vi "User Interface.vi"(8 "error in (no error)":errorcluster, 11 "User Interface in":refnum<class "User Interface.lvclass">) -> (0 "error out":errorcluster, 3 "User Interface out":refnum<class "User Interface.lvclass">)   [LabVIEW 2017, in "DSF Core.lvlib" / "Component Settings Editor.lvclass"]
uses:
  Component Settings Editor.lvclass
  User Interface.lvclass
  C:/Git/DSF/Core/Classes/User Interface/User Interface.lvclass
  Component Settings Editor.lvclass/Component Settings Editor.ctl
  User Interface Handler/User Interface Handler.lvclass
panel:
  in  "Components":i32(listbox)
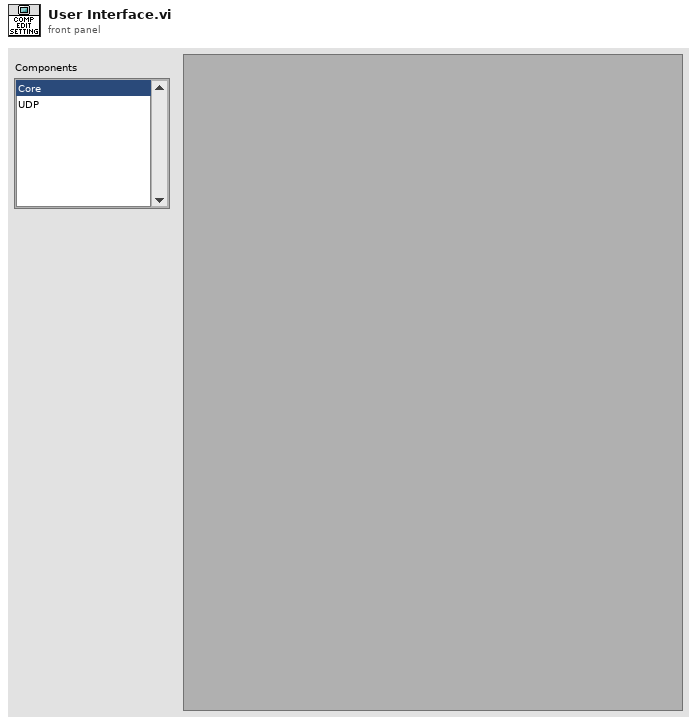
[diagram p1: front panel]
types:
  T1 = typedef "DSF Core.lvlib/User Interface Handler.lvclass/User Interface Ref.ctl" = refnum<vi>
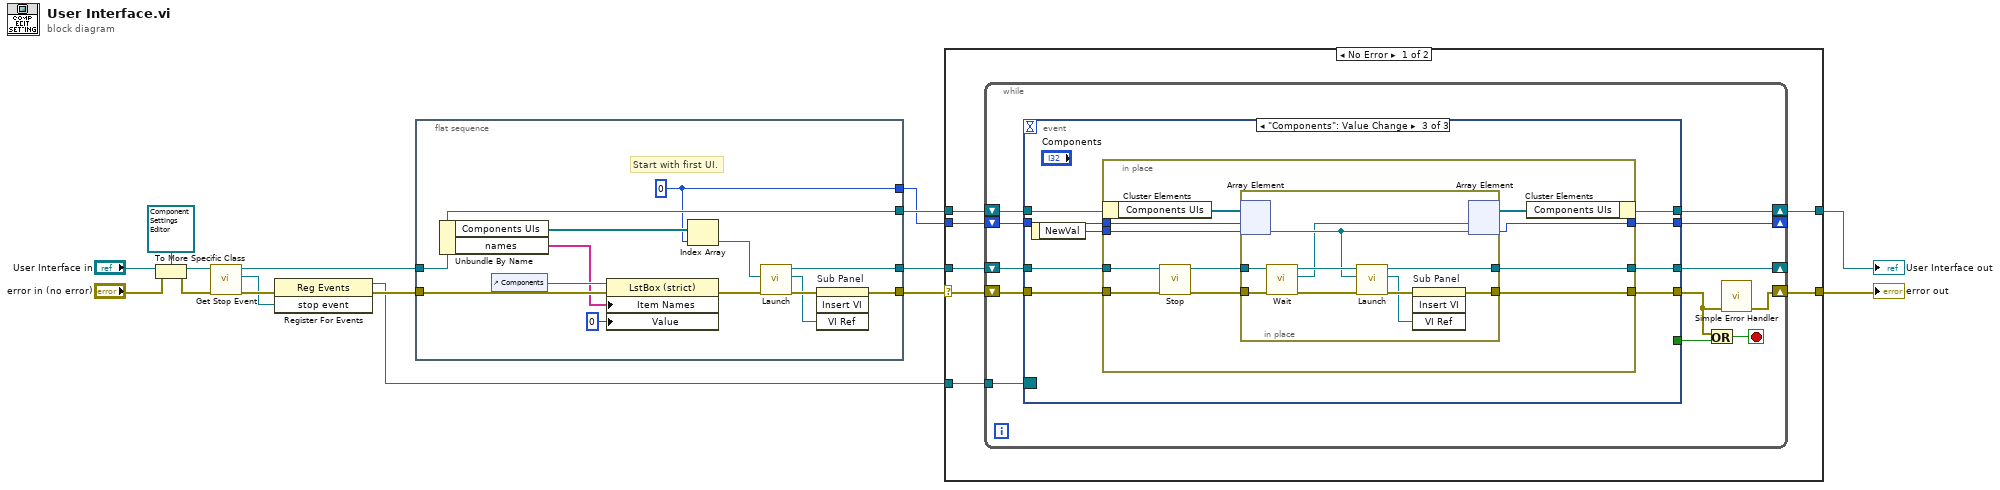
[diagram p0: block diagram]
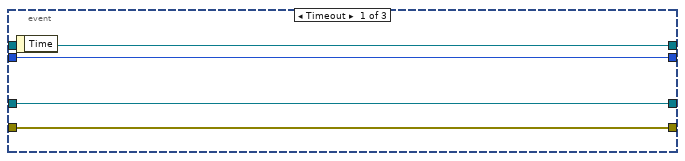
[diagram p2: hidden frame]
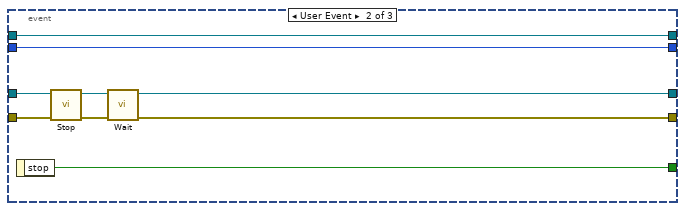
[diagram p3: hidden frame]
diagram:
  n1 = To More Specific Class(target class=refnum<class "Component Settings Editor.lvclass"> refnum ("DSF Core.lvlib:Plugin Settings Editor.lvclass"), reference="User Interface in", error in="error in (no error)") -> (specific class reference=w10:refnum<class "Component Settings Editor.lvclass">, error out=w9:errorcluster)
  n2 = call "Get Stop Event.vi"("error in (no error)"=w9, "User Interface in"=w10) -> ("error out"=w12:errorcluster, "stop event"=w11:refnum<user-event>, "User Interface out"=w4:refnum<class "Component Settings Editor.lvclass">)  [unwired: 7 in]
  n3 = register-events(error in=w12, w11) -> (reference out=w6:refnum<event-registration>, error out=w7:errorcluster)  [unwired: 1 in]
  n4 = flat-sequence {
    tunnel: w7 -> [w28]
    tunnel: [w25] -> w1
    tunnel: [w23] -> w5
    tunnel: w4 -> [w22]
    tunnel: [w22] -> w3
    tunnel: [w17] -> w2
    frame #0 {
      w17 = 0
      # "Start with first UI."
      n5 = Unbundle By Name(w22) -> ("Components UIs"=w21:refnum<class "User Interface.lvclass">[], "names"=w20:string[])
      n6 = control-ref of="Components"() -> (w29:refnum<vi>)
      n7 = property class="LstBox (strict)"(reference=w29, error in=w28, "Item Names"=w20, "Value"=0) -> (error out=w18:errorcluster)  [unwired: 1 out]
      n8 = Index Array(array=w21, index=w17) -> (element=w19:refnum<class "User Interface.lvclass">)
      n9 = call "Launch.vi"("error in (no error)"=w18, "User Interface"=w19) -> ("error out"=w26:errorcluster, "active vi"=w24:T1, "User Interface Handler out"=w23:refnum<class "User Interface Handler.lvclass">)  [unwired: 7 in]
      n10 = invoke on="Sub Panel" class="SubPnl" method="Insert VI"(error in=w26, "VI Ref"=w24) -> (error out=w25:errorcluster)  [unwired: 2 in, 3 out]
    }
  }
  n11 = case shown="No Error" w1 {
    selector: w1 -> [w30 w93]
    tunnel: [w36 w93] -> w16
    tunnel: [w35 w92] -> w13
    tunnel: w6 -> [w34 _]
    tunnel: w5 -> [w33 _]
    tunnel: w3 -> [w32 w92]
    tunnel: w2 -> [w31 _]
    frame No Error {
      n12 = while {
        tunnel: w34 -> [w48]
        shift-right: [w37] -> w36
        shift-left: w30 -> [w47]
        shift-right: [w43] -> _
        shift-left: w33 -> [w44]
        shift-right: [w41] -> w35
        shift-left: w32 -> [w42]
        shift-right: [w39] -> _
        shift-left: w31 -> [w40]
        stop <- w46 stop-if-true
        n13 = event shown="[2] \"Components\": Value Change" {
          selector: w48 -> [_ _ _]
          dyn-events: _ -> [_ _ _]
          timeout: _ -> [_ _ _]
          tunnel: [_ w61 _] -> w45
          tunnel: w47 -> [w52 w57 w65]
          tunnel: [w52 w56 w62] -> w38
          tunnel: w44 -> [w51 w58 w64]
          tunnel: [w51 w55 w63] -> w43
          tunnel: w42 -> [w50 w54 w70]
          tunnel: [w50 w54 w69] -> w41
          tunnel: w40 -> [w49 w53 w67]
          tunnel: [w49 w53 w66] -> w39
          event Timeout {
            n14 = event-data() -> ()  [unwired: 1 in, 1 out]
          }
          event User Event {
            n15 = event-data() -> ("stop"=w61:bool)  [unwired: 1 in]
            n16 = call "Stop.vi"("error in (no error)"=w57, "User Interface Handler in"=w58) -> ("error out"=w59:errorcluster, "User Interface Handler out"=w60:refnum<class "User Interface Handler.lvclass">)  [unwired: 8 in]
            n17 = call "Wait.vi"("error in (no error)"=w59, "User Interface Handler in"=w60) -> ("error out"=w56:errorcluster, "User Interface Handler out"=w55:refnum<class "User Interface Handler.lvclass">)  [unwired: 7 in, 1 out]
          }
          event "Components": Value Change {
            n18 = event-data() -> ("NewVal"=w68:i32)  [unwired: 1 in]
            n19 = in-place {
              in-place-border: w67 -> [w81]
              in-place-border: w68 -> [w77]
              in-place-border: [w80] -> w66
              in-place-border: w65 -> [w73]
              in-place-border: w64 -> [w74]
              in-place-border: [w79] -> w63
              in-place-border: [w78] -> w62
              n20 = in-place-cluster #1(w70) -> ("Components UIs"=w76:refnum<class "User Interface.lvclass">[])
              n21 = call "Stop.vi"("error in (no error)"=w73, "User Interface Handler in"=w74) -> ("error out"=w72:errorcluster, "User Interface Handler out"=w71:refnum<class "User Interface Handler.lvclass">)  [unwired: 8 in]
              n22 = in-place {
                in-place-border: [w89] -> w79
                in-place-border: [w90] -> w78
                in-place-border: w72 -> [w83]
                in-place-border: w71 -> [w82]
                n23 = in-place-array #2(w76, w81, w77) -> (w85:refnum<class "User Interface.lvclass">)  [unwired: 1 out]
                n24 = call "Wait.vi"("error in (no error)"=w83, "User Interface Handler in"=w82) -> ("error out"=w87:errorcluster, "User Interface"=w84:refnum<class "User Interface.lvclass">, "User Interface Handler out"=w86:refnum<class "User Interface Handler.lvclass">)  [unwired: 7 in]
                n25 = call "Launch.vi"("error in (no error)"=w87, "User Interface"=w85, "User Interface Handler in"=w86) -> ("error out"=w91:errorcluster, "active vi"=w88:T1, "User Interface Handler out"=w89:refnum<class "User Interface Handler.lvclass">)  [unwired: 6 in]
                n26 = invoke on="Sub Panel" class="SubPnl" method="Insert VI"(error in=w91, "VI Ref"=w88) -> (error out=w90:errorcluster)  [unwired: 2 in, 3 out]
                n27 = in-place-array #2(w84, w85) -> (w75:refnum<class "User Interface.lvclass">[], w80:i32)  [unwired: 1 out]
              }
              n28 = in-place-cluster #1("Components UIs"=w75) -> (w69:refnum<class "Component Settings Editor.lvclass">)
            }
          }
        }
        n29 = Or(x=w38, y=w45) -> (x .or. y?=w46:bool)
        n30 = call <vilib>:"Simple Error Handler.vi"("error in (no error)"=w38) -> ("error out"=w37:errorcluster)  [unwired: 4 in, 4 out]
      }
    }
    frame Error {
    }
  }
  "error out" <- w16
  "User Interface out" <- w13
